vi "Open_Instr.vi"(8 "error in (no error)":errorcluster caption="entrée d'erreur (pas d'erreur)", 11 "Class Multimeter Multimeter en entrée":refnum<class "Class Instrument Balance.lvclass">) -> (0 "error out":errorcluster caption="sortie d'erreur", 3 "Class Multimeter Multimeter en sortie":refnum<class "Class Instrument Balance.lvclass">)   [LabVIEW 2020, in "Library Instrument & Equipement.lvlib" / "Library Instruments.lvlib" / "Class Instrument Balance.lvclass"]
uses:
  Class Instrument Balance.lvclass
  Class Instrument Balance.lvclass/Class Instrument Balance.ctl
  Instrument (Default)/Class Instrument (Default).lvclass
  Balance/Balance (Default)/Class Balance (Default).lvclass
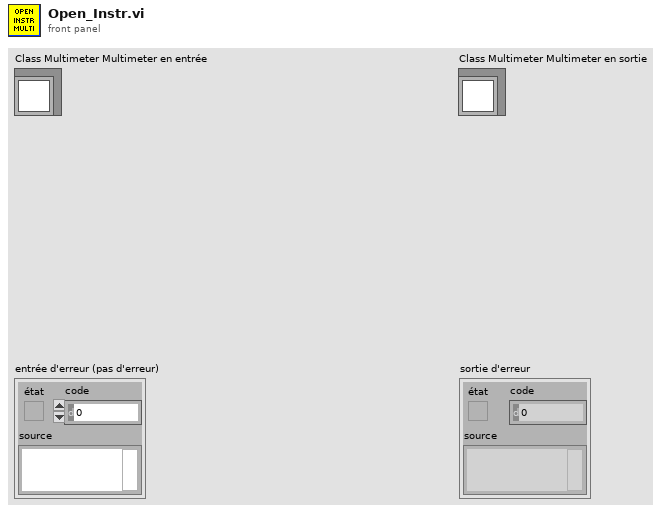
[diagram p1: front panel]
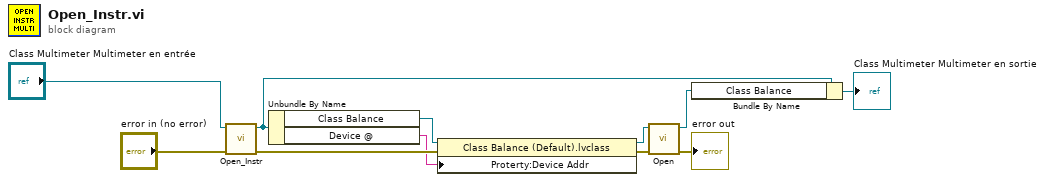
[diagram p0: block diagram]
diagram:
  n1 = call-parent "Open_Instr.vi"("error in (no error)"="error in (no error)", "Class Multimeter (Default) en entrée"="Class Multimeter Multimeter en entrée") -> ("error out"=w8:errorcluster, "Class Multimeter (Default) en sortie"=w5:refnum<class "Class Instrument Balance.lvclass">)  [unwired: 8 in]
  n2 = Unbundle By Name(w5) -> ("Class Balance"=w9:refnum<class "Class Balance (Default).lvclass">, "Device @"=w7:string)
  n3 = property class="Class Balance (Default).lvclass"(reference=w9, error in=w8, "Proterty:Device Addr"=w7) -> (reference out=w3:refnum<class "Class Balance (Default).lvclass">, error out=w4:errorcluster)
  n4 = call-dynamic "Open.vi"("error in (no error)"=w4, "Class Balance (Default) en entrée"=w3) -> ("error out"=→"error out":errorcluster, "Class Balance (Default) en sortie"=w2:refnum<class "Class Balance (Default).lvclass">)  [unwired: 8 in]
  n5 = Bundle By Name(cluster=w5, "Class Balance"=w2) -> (→"Class Multimeter Multimeter en sortie":refnum<class "Class Instrument Balance.lvclass">)
